vi "PicoScopeospaSettings.vi"(0 "handle in":i16=16384, 1 "Device Info":T3={"PICO_DRIVER_VERSION"="", "PICO_USB_VERSION"="", "PICO_HARDWARE_VERSION"="", "PICO_VARIANT_INFO"="", "PICO_BATCH_AND_SERIAL"="", "PICO_CAL_DATE"="", "PICO_KERNEL_VERSION"="", "PICO_DIGITAL_HARDWARE_VERSION"="", "PICO_ANALOGUE_HARDWARE_VERSION"="", "PICO_FIRMWARE_VERSION_1"="", "PICO_FIRMWARE_VERSION_2"="", "PICO_IPP_VERSION"="", "PICO_DRIVER_PATH"="", "PICO_FIRMWARE_VERSION_3"="", "PICO_FRONT_PANEL_FIRMWARE_VERSION"="", "Number of Channels"=0, "MSO"=TRUE}, 2 "Channels":T2={"Channel A Settings "={"Enabled"=FALSE, "Coupling"=1, "Range"=8, "Analogue Offset"=0.0, "BandWidth"=0, "PROBE_RANGE_INFO"=0}, "Channel B Settings "={"Enabled"=FALSE, "Coupling"=1, "Range"=8, "Analogue Offset"=0.0, "BandWidth"=0, "PROBE_RANGE_INFO"=0}, "Channel C Settings "={"Enabled"=FALSE, "Coupling"=1, "Range"=8, "Analogue Offset"=0.0, "BandWidth"=0, "PROBE_RANGE_INFO"=0}, "Channel D Settings "={"Enabled"=FALSE, "Coupling"=1, "Range"=8, "Analogue Offset"=0.0, "BandWidth"=0, "PROBE_RANGE_INFO"=0}, "Channel E Settings "={"Enabled"=FALSE, "Coupling"=50, "Range"=5, "Analogue Offset"=0.0, "BandWidth"=0, "PROBE_RANGE_INFO"=0}, "Channel F Settings "={"Enabled"=FALSE, "Coupling"=50, "Range"=5, "Analogue Offset"=0.0, "BandWidth"=0, "PROBE_RANGE_INFO"=0}, "Channel G Settings "={"Enabled"=FALSE, "Coupling"=50, "Range"=5, "Analogue Offset"=0.0, "BandWidth"=0, "PROBE_RANGE_INFO"=0}, "Channel H Settings "={"Enabled"=FALSE, "Coupling"=50, "Range"=5, "Analogue Offset"=0.0, "BandWidth"=0, "PROBE_RANGE_INFO"=0}} {"Channel H Settings"."PROBE_RANGE_INFO" items=["PROBE_NONE_NV"=0, "X1_PROBE_NV"=1, "X10_PROBE_NV"=10]; "Channel H Settings"."BandWidth" items=["Full"=0, "100kHz"=100000, "20kHz"=200000, "1MHz"=1000000, "20MHz"=20000000, "25MHz"=25000000, "50MHz"=50000000, "200MHz"=200000000, "250MHz"=250000000, "500MHz"=500000000]; "Channel H Settings"."Range" items=["10mV"=0, "20mV"=1, "50mV"=2, "100mV"=3, "200mV"=4, "500mV"=5, "1V"=6, "2V"=7, "5V"=8, "10V"=9, "20V"=10, "50V"=11, "100V"=12, "200V"=13, "x10_Probe_100mV"=32, "x10_Probe_200mV"=33, "x10_Probe_500mV"=34, "x10_Probe_1V"=35, "x10_Probe_2V"=36, "x10_Probe_5V"=37, "x10_Probe_10V"=38, "x10_Probe_20V"=39, "x10_Probe_50V"=40, "x10_Probe_100V"=41, "x10_Probe_200V"=42, "x10_Probe_500V"=43, "CURRENT_CLAMP_60A_2A"=10500, "CURRENT_CLAMP_60A_5A"=10501, "CURRENT_CLAMP_60A_10A"=10502, "CURRENT_CLAMP_60A_20A"=10503, "CURRENT_CLAMP_60A_50A"=10504, "CURRENT_CLAMP_60A_60A"=10505, "CURRENT_CLAMP_60A_V2_0_5A"=10600, "CURRENT_CLAMP_60A_V2_1A"=10601, "CURRENT_CLAMP_60A_V2_2A"=10602, "CURRENT_CLAMP_60A_V2_5A"=10603, "CURRENT_CLAMP_60A_V2_10A"=10604, "CURRENT_CLAMP_60A_V2_20A"=10605, "CURRENT_CLAMP_60A_V2_50A"=10606, "CURRENT_CLAMP_60A_V2_60A"=10607, "RESISTANCE_LEAD_NEG5_TO_20OHM"=7000, "RESISTANCE_LEAD_NEG50_TO_200OHM"=7001, "RESISTANCE_LEAD_NEG500_TO_2KOHM"=7002, "RESISTANCE_LEAD_NEG5K_TO_20KOHM"=7003, "RESISTANCE_LEAD_NEG50K_TO_LEAD_200KOHM"=7004, "RESISTANCE_LEAD_NEG500K_TO_LEAD_2MOHM"=7005, "RESISTANCE_LEAD_DIODE_TEST"=7006, "HT_NEG3_TO_5KV"=8950, "HT_NEG3_TO_10KV"=8951, "HT_NEG5_TO_20KV"=8952, "HT_NEG5_TO_50KV"=8953, "HT_NEG5_TO_100KV"=8954, "HT_NEG3_TO_5KV_INVERTED"=8955, "HT_NEG3_TO_10KV_INVERTED"=8956, "HT_NEG5_TO_20KV_INVERTED"=8957, "HT_NEG5_TO_50KV_INVERTED"=8958, "HT_NEG5_TO_100KV_INVERTED"=8959, "TEMPERATURE_NEG50_TO_150DEGC"=9000, "PRESSURE_SENSOR_-100k-150k_PASCALS"=9100, "PRESSURE_SENSOR_-100k_TO_400k_PASCALS"=9101, "PRESSURE_SENSOR_-200k_TO_800k_PASCALS"=9102, "PRESSURE_SENSOR_-400k_TO_1600k_PASCALS"=9103, "PRESSURE_SENSOR_-400k_TO_3400k_PASCALS"=9104, "PRESSURE_SENSOR_-150k_TO_1350k_PASCALS"=9105]; "Channel H Settings"."Coupling" items=["AC"=0, "DC 1M Ohm"=1, "DC 50 Ohm"=50]; "Channel G Settings"."PROBE_RANGE_INFO" items=["PROBE_NONE_NV"=0, "X1_PROBE_NV"=1, "X10_PROBE_NV"=10]; "Channel G Settings"."BandWidth" items=["Full"=0, "100kHz"=100000, "20kHz"=200000, "1MHz"=1000000, "20MHz"=20000000, "25MHz"=25000000, "50MHz"=50000000, "200MHz"=200000000, "250MHz"=250000000, "500MHz"=500000000]; "Channel G Settings"."Range" items=["10mV"=0, "20mV"=1, "50mV"=2, "100mV"=3, "200mV"=4, "500mV"=5, "1V"=6, "2V"=7, "5V"=8, "10V"=9, "20V"=10, "50V"=11, "100V"=12, "200V"=13, "x10_Probe_100mV"=32, "x10_Probe_200mV"=33, "x10_Probe_500mV"=34, "x10_Probe_1V"=35, "x10_Probe_2V"=36, "x10_Probe_5V"=37, "x10_Probe_10V"=38, "x10_Probe_20V"=39, "x10_Probe_50V"=40, "x10_Probe_100V"=41, "x10_Probe_200V"=42, "x10_Probe_500V"=43, "CURRENT_CLAMP_60A_2A"=10500, "CURRENT_CLAMP_60A_5A"=10501, "CURRENT_CLAMP_60A_10A"=10502, "CURRENT_CLAMP_60A_20A"=10503, "CURRENT_CLAMP_60A_50A"=10504, "CURRENT_CLAMP_60A_60A"=10505, "CURRENT_CLAMP_60A_V2_0_5A"=10600, "CURRENT_CLAMP_60A_V2_1A"=10601, "CURRENT_CLAMP_60A_V2_2A"=10602, "CURRENT_CLAMP_60A_V2_5A"=10603, "CURRENT_CLAMP_60A_V2_10A"=10604, "CURRENT_CLAMP_60A_V2_20A"=10605, "CURRENT_CLAMP_60A_V2_50A"=10606, "CURRENT_CLAMP_60A_V2_60A"=10607, "RESISTANCE_LEAD_NEG5_TO_20OHM"=7000, "RESISTANCE_LEAD_NEG50_TO_200OHM"=7001, "RESISTANCE_LEAD_NEG500_TO_2KOHM"=7002, "RESISTANCE_LEAD_NEG5K_TO_20KOHM"=7003, "RESISTANCE_LEAD_NEG50K_TO_LEAD_200KOHM"=7004, "RESISTANCE_LEAD_NEG500K_TO_LEAD_2MOHM"=7005, "RESISTANCE_LEAD_DIODE_TEST"=7006, "HT_NEG3_TO_5KV"=8950, "HT_NEG3_TO_10KV"=8951, "HT_NEG5_TO_20KV"=8952, "HT_NEG5_TO_50KV"=8953, "HT_NEG5_TO_100KV"=8954, "HT_NEG3_TO_5KV_INVERTED"=8955, "HT_NEG3_TO_10KV_INVERTED"=8956, "HT_NEG5_TO_20KV_INVERTED"=8957, "HT_NEG5_TO_50KV_INVERTED"=8958, "HT_NEG5_TO_100KV_INVERTED"=8959, "TEMPERATURE_NEG50_TO_150DEGC"=9000, "PRESSURE_SENSOR_-100k-150k_PASCALS"=9100, "PRESSURE_SENSOR_-100k_TO_400k_PASCALS"=9101, "PRESSURE_SENSOR_-200k_TO_800k_PASCALS"=9102, "PRESSURE_SENSOR_-400k_TO_1600k_PASCALS"=9103, "PRESSURE_SENSOR_-400k_TO_3400k_PASCALS"=9104, "PRESSURE_SENSOR_-150k_TO_1350k_PASCALS"=9105]; "Channel G Settings"."Coupling" items=["AC"=0, "DC 1M Ohm"=1, "DC 50 Ohm"=50]; "Channel F Settings"."PROBE_RANGE_INFO" items=["PROBE_NONE_NV"=0, "X1_PROBE_NV"=1, "X10_PROBE_NV"=10]; "Channel F Settings"."BandWidth" items=["Full"=0, "100kHz"=100000, "20kHz"=200000, "1MHz"=1000000, "20MHz"=20000000, "25MHz"=25000000, "50MHz"=50000000, "200MHz"=200000000, "250MHz"=250000000, "500MHz"=500000000]; "Channel F Settings"."Range" items=["10mV"=0, "20mV"=1, "50mV"=2, "100mV"=3, "200mV"=4, "500mV"=5, "1V"=6, "2V"=7, "5V"=8, "10V"=9, "20V"=10, "50V"=11, "100V"=12, "200V"=13, "x10_Probe_100mV"=32, "x10_Probe_200mV"=33, "x10_Probe_500mV"=34, "x10_Probe_1V"=35, "x10_Probe_2V"=36, "x10_Probe_5V"=37, "x10_Probe_10V"=38, "x10_Probe_20V"=39, "x10_Probe_50V"=40, "x10_Probe_100V"=41, "x10_Probe_200V"=42, "x10_Probe_500V"=43, "CURRENT_CLAMP_60A_2A"=10500, "CURRENT_CLAMP_60A_5A"=10501, "CURRENT_CLAMP_60A_10A"=10502, "CURRENT_CLAMP_60A_20A"=10503, "CURRENT_CLAMP_60A_50A"=10504, "CURRENT_CLAMP_60A_60A"=10505, "CURRENT_CLAMP_60A_V2_0_5A"=10600, "CURRENT_CLAMP_60A_V2_1A"=10601, "CURRENT_CLAMP_60A_V2_2A"=10602, "CURRENT_CLAMP_60A_V2_5A"=10603, "CURRENT_CLAMP_60A_V2_10A"=10604, "CURRENT_CLAMP_60A_V2_20A"=10605, "CURRENT_CLAMP_60A_V2_50A"=10606, "CURRENT_CLAMP_60A_V2_60A"=10607, "RESISTANCE_LEAD_NEG5_TO_20OHM"=7000, "RESISTANCE_LEAD_NEG50_TO_200OHM"=7001, "RESISTANCE_LEAD_NEG500_TO_2KOHM"=7002, "RESISTANCE_LEAD_NEG5K_TO_20KOHM"=7003, "RESISTANCE_LEAD_NEG50K_TO_LEAD_200KOHM"=7004, "RESISTANCE_LEAD_NEG500K_TO_LEAD_2MOHM"=7005, "RESISTANCE_LEAD_DIODE_TEST"=7006, "HT_NEG3_TO_5KV"=8950, "HT_NEG3_TO_10KV"=8951, "HT_NEG5_TO_20KV"=8952, "HT_NEG5_TO_50KV"=8953, "HT_NEG5_TO_100KV"=8954, "HT_NEG3_TO_5KV_INVERTED"=8955, "HT_NEG3_TO_10KV_INVERTED"=8956, "HT_NEG5_TO_20KV_INVERTED"=8957, "HT_NEG5_TO_50KV_INVERTED"=8958, "HT_NEG5_TO_100KV_INVERTED"=8959, "TEMPERATURE_NEG50_TO_150DEGC"=9000, "PRESSURE_SENSOR_-100k-150k_PASCALS"=9100, "PRESSURE_SENSOR_-100k_TO_400k_PASCALS"=9101, "PRESSURE_SENSOR_-200k_TO_800k_PASCALS"=9102, "PRESSURE_SENSOR_-400k_TO_1600k_PASCALS"=9103, "PRESSURE_SENSOR_-400k_TO_3400k_PASCALS"=9104, "PRESSURE_SENSOR_-150k_TO_1350k_PASCALS"=9105]; "Channel F Settings"."Coupling" items=["AC"=0, "DC 1M Ohm"=1, "DC 50 Ohm"=50]; "Channel E Settings"."PROBE_RANGE_INFO" items=["PROBE_NONE_NV"=0, "X1_PROBE_NV"=1, "X10_PROBE_NV"=10]; "Channel E Settings"."BandWidth" items=["Full"=0, "100kHz"=100000, "20kHz"=200000, "1MHz"=1000000, "20MHz"=20000000, "25MHz"=25000000, "50MHz"=50000000, "200MHz"=200000000, "250MHz"=250000000, "500MHz"=500000000]; "Channel E Settings"."Range" items=["10mV"=0, "20mV"=1, "50mV"=2, "100mV"=3, "200mV"=4, "500mV"=5, "1V"=6, "2V"=7, "5V"=8, "10V"=9, "20V"=10, "50V"=11, "100V"=12, "200V"=13, "x10_Probe_100mV"=32, "x10_Probe_200mV"=33, "x10_Probe_500mV"=34, "x10_Probe_1V"=35, "x10_Probe_2V"=36, "x10_Probe_5V"=37, "x10_Probe_10V"=38, "x10_Probe_20V"=39, "x10_Probe_50V"=40, "x10_Probe_100V"=41, "x10_Probe_200V"=42, "x10_Probe_500V"=43, "CURRENT_CLAMP_60A_2A"=10500, "CURRENT_CLAMP_60A_5A"=10501, "CURRENT_CLAMP_60A_10A"=10502, "CURRENT_CLAMP_60A_20A"=10503, "CURRENT_CLAMP_60A_50A"=10504, "CURRENT_CLAMP_60A_60A"=10505, "CURRENT_CLAMP_60A_V2_0_5A"=10600, "CURRENT_CLAMP_60A_V2_1A"=10601, "CURRENT_CLAMP_60A_V2_2A"=10602, "CURRENT_CLAMP_60A_V2_5A"=10603, "CURRENT_CLAMP_60A_V2_10A"=10604, "CURRENT_CLAMP_60A_V2_20A"=10605, "CURRENT_CLAMP_60A_V2_50A"=10606, "CURRENT_CLAMP_60A_V2_60A"=10607, "RESISTANCE_LEAD_NEG5_TO_20OHM"=7000, "RESISTANCE_LEAD_NEG50_TO_200OHM"=7001, "RESISTANCE_LEAD_NEG500_TO_2KOHM"=7002, "RESISTANCE_LEAD_NEG5K_TO_20KOHM"=7003, "RESISTANCE_LEAD_NEG50K_TO_LEAD_200KOHM"=7004, "RESISTANCE_LEAD_NEG500K_TO_LEAD_2MOHM"=7005, "RESISTANCE_LEAD_DIODE_TEST"=7006, "HT_NEG3_TO_5KV"=8950, "HT_NEG3_TO_10KV"=8951, "HT_NEG5_TO_20KV"=8952, "HT_NEG5_TO_50KV"=8953, "HT_NEG5_TO_100KV"=8954, "HT_NEG3_TO_5KV_INVERTED"=8955, "HT_NEG3_TO_10KV_INVERTED"=8956, "HT_NEG5_TO_20KV_INVERTED"=8957, "HT_NEG5_TO_50KV_INVERTED"=8958, "HT_NEG5_TO_100KV_INVERTED"=8959, "TEMPERATURE_NEG50_TO_150DEGC"=9000, "PRESSURE_SENSOR_-100k-150k_PASCALS"=9100, "PRESSURE_SENSOR_-100k_TO_400k_PASCALS"=9101, "PRESSURE_SENSOR_-200k_TO_800k_PASCALS"=9102, "PRESSURE_SENSOR_-400k_TO_1600k_PASCALS"=9103, "PRESSURE_SENSOR_-400k_TO_3400k_PASCALS"=9104, "PRESSURE_SENSOR_-150k_TO_1350k_PASCALS"=9105]; "Channel E Settings"."Coupling" items=["AC"=0, "DC 1M Ohm"=1, "DC 50 Ohm"=50]; "Channel D Settings"."BandWidth" items=["Full"=0, "100kHz"=100000, "20kHz"=200000, "1MHz"=1000000, "20MHz"=20000000, "25MHz"=25000000, "50MHz"=50000000, "100MHz"=100000000, "200MHz"=200000000, "250MHz"=250000000, "350MHz"=350000000, "500MHz"=500000000]; "Channel D Settings"."PROBE_RANGE_INFO" items=["PROBE_NONE_NV"=0, "X1_PROBE_NV"=1, "X10_PROBE_NV"=10]; "Channel D Settings"."Range" items=["10mV", "20mV", "50mV", "100mV", "200mV", "500mV", "1V", "2V", "5V", "10V", "20V", "50V", "100V", "200V"]; "Channel D Settings"."Coupling" items=["AC"=0, "DC 1M Ohm"=1, "DC 50 Ohm"=50]; "Channel C Settings"."BandWidth" items=["Full"=0, "100kHz"=100000, "20kHz"=200000, "1MHz"=1000000, "20MHz"=20000000, "25MHz"=25000000, "50MHz"=50000000, "100MHz"=100000000, "200MHz"=200000000, "250MHz"=250000000, "350MHz"=350000000, "500MHz"=500000000]; "Channel C Settings"."PROBE_RANGE_INFO" items=["PROBE_NONE_NV"=0, "X1_PROBE_NV"=1, "X10_PROBE_NV"=10]; "Channel C Settings"."Range" items=["10mV", "20mV", "50mV", "100mV", "200mV", "500mV", "1V", "2V", "5V", "10V", "20V", "50V", "100V", "200V"]; "Channel C Settings"."Coupling" items=["AC"=0, "DC 1M Ohm"=1, "DC 50 Ohm"=50]; "Channel B Settings"."BandWidth" items=["Full"=0, "100kHz"=100000, "20kHz"=200000, "1MHz"=1000000, "20MHz"=20000000, "25MHz"=25000000, "50MHz"=50000000, "100MHz"=100000000, "200MHz"=200000000, "250MHz"=250000000, "350MHz"=350000000, "500MHz"=500000000]; "Channel B Settings"."PROBE_RANGE_INFO" items=["PROBE_NONE_NV"=0, "X1_PROBE_NV"=1, "X10_PROBE_NV"=10]; "Channel B Settings"."Range" items=["10mV", "20mV", "50mV", "100mV", "200mV", "500mV", "1V", "2V", "5V", "10V", "20V", "50V", "100V", "200V"]; "Channel B Settings"."Coupling" items=["AC"=0, "DC 1M Ohm"=1, "DC 50 Ohm"=50]; "Channel A Settings"."PROBE_RANGE_INFO" items=["PROBE_NONE_NV"=0, "X1_PROBE_NV"=1, "X10_PROBE_NV"=10]; "Channel A Settings"."Range" items=["10mV", "20mV", "50mV", "100mV", "200mV", "500mV", "1V", "2V", "5V", "10V", "20V", "50V", "100V", "200V"]; "Channel A Settings"."BandWidth" items=["Full"=0, "100kHz"=100000, "20kHz"=200000, "1MHz"=1000000, "20MHz"=20000000, "25MHz"=25000000, "50MHz"=50000000, "100MHz"=100000000, "200MHz"=200000000, "250MHz"=250000000, "350MHz"=350000000, "500MHz"=500000000]; "Channel A Settings"."Coupling" items=["AC"=0, "DC 1M Ohm"=1, "DC 50 Ohm"=50]}, 7 "Max ADC value":i16=32512, 11 "error in (no error)":errorcluster, 12 "Trigger Settings":T4={"Trigger Enabled"=FALSE, "Trigger Threshold (Volts/Probe Units)"=0.0, "Trigger Direction"=2, "Trigger Delay (samples)"=0, "Auto Trigger Time (us)"=1000000, "Trigger Source"=0} {"Trigger Source" items=["Channel A"=0, "Channel B"=1, "Channel C"=2, "Channel D"=3, "Channel E"=4, "Channel F"=5, "Channel G"=6, "Channel H"=7, "Port 0"=128, "Port 1"=129, "Trigger AUX"=1001]; "Trigger Direction" items=["Above", "Below", "Rising", "Falling", "Rising or Falling"]; "Trigger Threshold (Volts/Probe Units)" format="%#_6p"}, 14 "Digital Channels":T1 {"Port 1 Settings"."Threshold Level (Volts)" format="%#_4p"; "Port 0 Settings"."Threshold Level (Volts)" format="%#_4p"}) -> (3 "Enabled array":i16[](array[numeric])=[1, 0, 0, 0, 0, 0, 0, 0, 0, 0], 4 "handle out":i16=16384, 15 "error out":errorcluster)   [LabVIEW 2024]
doc: "Sets up channels and calls setSimpleTrigger"
uses:
  PicoScopeospaAnalogChannelSettings.ctl
  PicoScopeospaDigitalChannelSettings.ctl
  psospa.dll
panel:
  # "D8-D15"
  # "DO-D7"
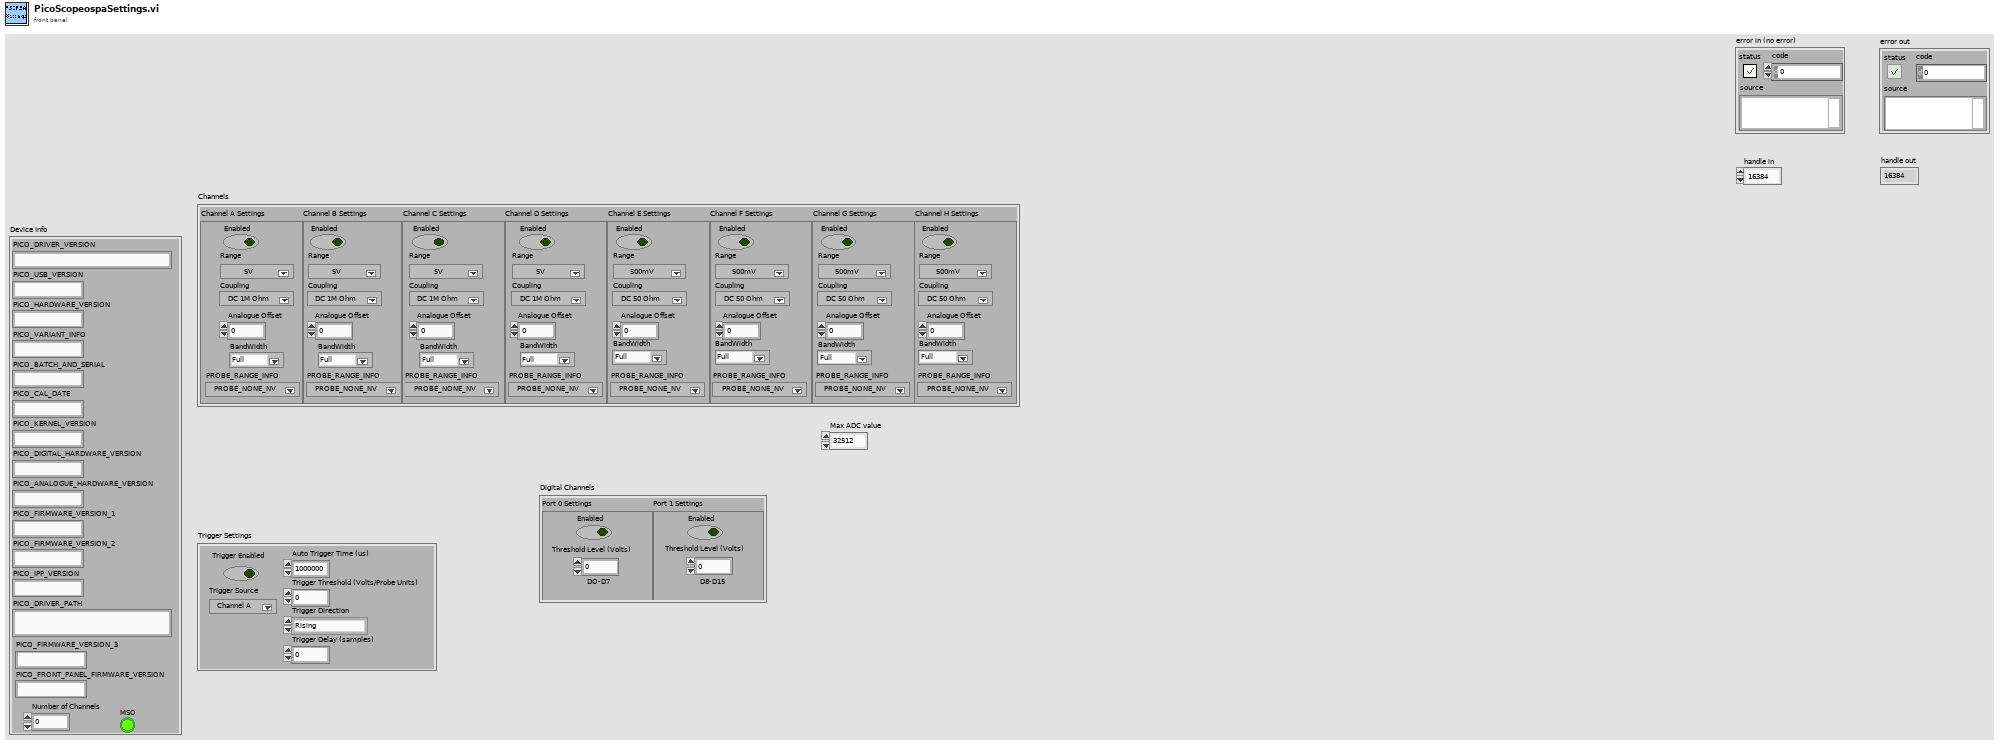
[diagram p1: front panel]
types:
  T1 = typedef "PicoScopeospaDigitalChannelSettings.ctl" = cluster{"Port 0 Settings ":cluster{"Enabled":bool, "Threshold Level (Volts)":dbl}, "Port 1 Settings":cluster{"Enabled":bool, "Threshold Level (Volts)":dbl}}
  T2 = typedef "PicoScopeospaAnalogChannelSettings.ctl" = cluster{"Channel A Settings ":cluster{"Enabled":bool, "Coupling":i16, "Range":u16, "Analogue Offset":dbl, "BandWidth":u32, "PROBE_RANGE_INFO":u32}, "Channel B Settings ":cluster{"Enabled":bool, "Coupling":i16, "Range":u16, "Analogue Offset":dbl, "BandWidth":u32, "PROBE_RANGE_INFO":u32}, "Channel C Settings ":cluster{"Enabled":bool, "Coupling":i16, "Range":u16, "Analogue Offset":dbl, "BandWidth":u32, "PROBE_RANGE_INFO":u32}, "Channel D Settings ":cluster{"Enabled":bool, "Coupling":i16, "Range":u16, "Analogue Offset":dbl, "BandWidth":u32, "PROBE_RANGE_INFO":u32}, "Channel E Settings ":cluster{"Enabled":bool, "Coupling":i16, "Range":u16, "Analogue Offset":dbl, "BandWidth":u32, "PROBE_RANGE_INFO":u32}, "Channel F Settings ":cluster{"Enabled":bool, "Coupling":i16, "Range":u16, "Analogue Offset":dbl, "BandWidth":u32, "PROBE_RANGE_INFO":u32}, "Channel G Settings ":cluster{"Enabled":bool, "Coupling":i16, "Range":u16, "Analogue Offset":dbl, "BandWidth":u32, "PROBE_RANGE_INFO":u32}, "Channel H Settings ":cluster{"Enabled":bool, "Coupling":i16, "Range":u16, "Analogue Offset":dbl, "BandWidth":u32, "PROBE_RANGE_INFO":u32}}
  T3 = cluster{"PICO_DRIVER_VERSION":string, "PICO_USB_VERSION":string, "PICO_HARDWARE_VERSION":string, "PICO_VARIANT_INFO":string, "PICO_BATCH_AND_SERIAL":string, "PICO_CAL_DATE":string, "PICO_KERNEL_VERSION":string, "PICO_DIGITAL_HARDWARE_VERSION":string, "PICO_ANALOGUE_HARDWARE_VERSION":string, "PICO_FIRMWARE_VERSION_1":string, "PICO_FIRMWARE_VERSION_2":string, "PICO_IPP_VERSION":string, "PICO_DRIVER_PATH":string, "PICO_FIRMWARE_VERSION_3":string, "PICO_FRONT_PANEL_FIRMWARE_VERSION":string, "Number of Channels":i16, "MSO":bool}
  T4 = cluster{"Trigger Enabled":bool, "Trigger Threshold (Volts/Probe Units)":dbl, "Trigger Direction":u16, "Trigger Delay (samples)":u64, "Auto Trigger Time (us)":u32, "Trigger Source":u32}
  T5 = cluster{"Enabled":bool, "Coupling":i16, "Range":u16, "Analogue Offset":dbl, "BandWidth":u32, "PROBE_RANGE_INFO":u32}
  T6 = cluster{"Enabled":bool, "Threshold Level (Volts)":dbl}
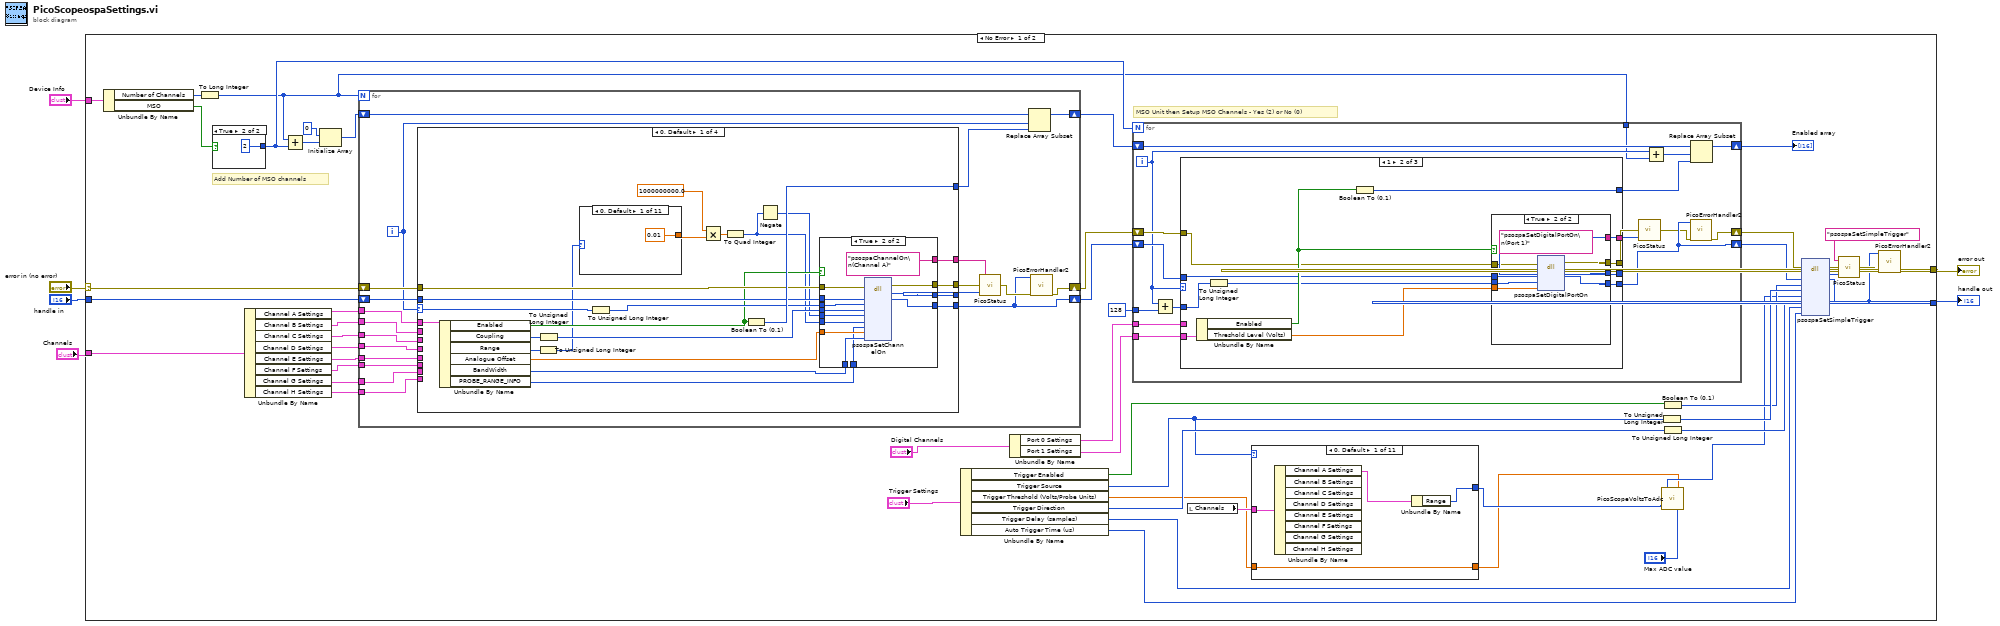
[diagram p0: block diagram]
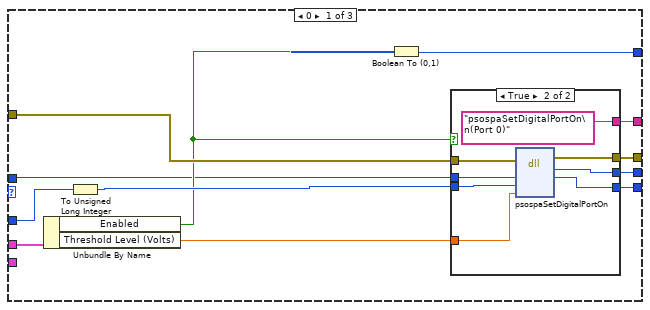
[diagram p2: hidden frame]
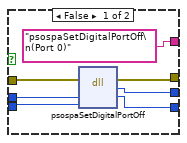
[diagram p3: hidden frame]
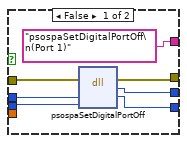
[diagram p4: hidden frame]
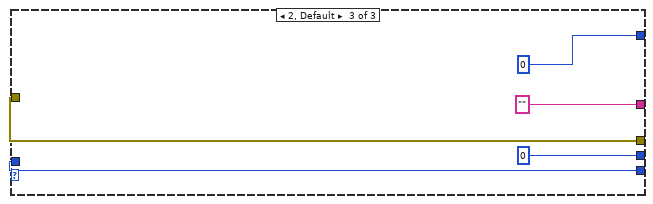
[diagram p5: hidden frame]
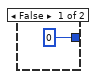
[diagram p6: hidden frame]
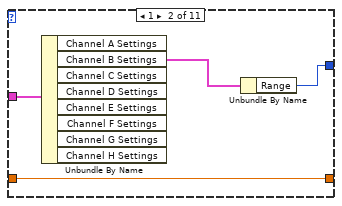
[diagram p7: hidden frame]
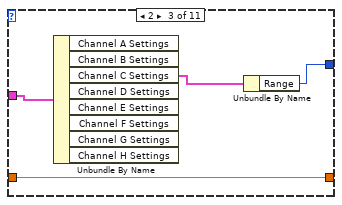
[diagram p8: hidden frame]
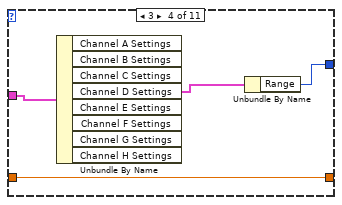
[diagram p9: hidden frame]
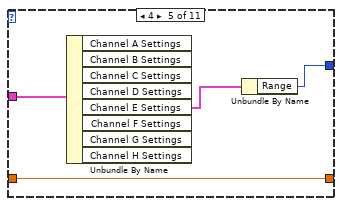
[diagram p10: hidden frame]
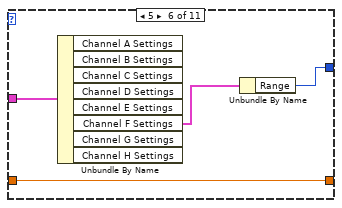
[diagram p11: hidden frame]
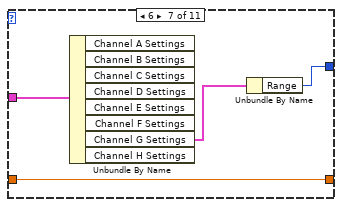
[diagram p12: hidden frame]
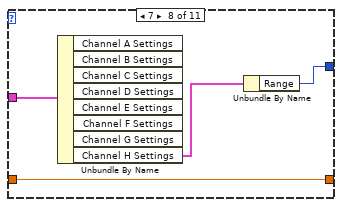
[diagram p13: hidden frame]
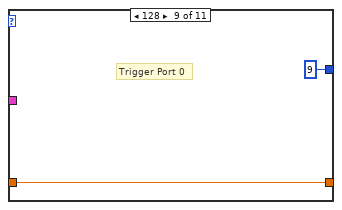
[diagram p14: hidden frame]
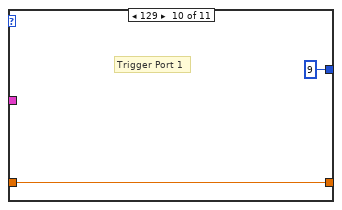
[diagram p15: hidden frame]
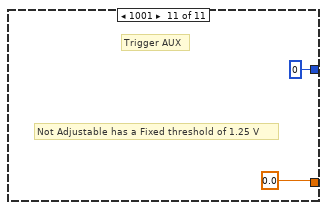
[diagram p16: hidden frame]
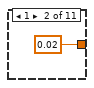
[diagram p17: hidden frame]
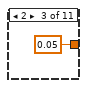
[diagram p18: hidden frame]
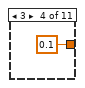
[diagram p19: hidden frame]
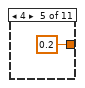
[diagram p20: hidden frame]
diagram:
  n1 = case shown="No Error" "error in (no error)" {
    selector: "error in (no error)" -> [w44 w411]
    tunnel: "handle in" -> [w45 w410]
    tunnel: [w37 w410] -> w6
    tunnel: [w39 w411] -> w5
    tunnel: "Device Info" -> [w41 _]
    tunnel: "Channels" -> [w28 _]
    frame No Error {
      # "Add Number of MSO channels"
      # "MSO Unit then Setup MSO Channels - Yes (2) or No (0)"
      n2 = Unbundle By Name(w41) -> ("Number of Channels"=w40:i16, "MSO"=w11:bool)
      n3 = To Long Integer(number=w40) -> (32bit integer=w8:i32)
      n4 = case shown="True" w11 {
        tunnel: [0 ("y") 2 ("y")] -> w9
        frame False {
        }
        frame True {
        }
      }
      n5 = Unbundle By Name(w28) -> ("Channel A Settings"=w35:T5, "Channel B Settings"=w36:T5, "Channel C Settings"=w34:T5, "Channel D Settings"=w33:T5, "Channel E Settings"=w32:T5, "Channel F Settings"=w29:T5, "Channel G Settings"=w30:T5, "Channel H Settings"=w31:T5)
      n6 = Add(x=w8, y=w9) -> (x+y=w12:i32)
      n7 = Initialize Array(i16 0 ("element"), w12) -> (w42:i16[])
      n8 = for {
        N: w8 -> [_]
        shift-right: [w187] -> w24
        shift-left: w44 -> [w192]
        shift-right: [w182] -> w23
        shift-left: w45 -> [w193]
        shift-right: [w188] -> w26
        shift-left: w42 -> [w189]
        tunnel: w36 -> [w181]
        tunnel: w35 -> [w180]
        tunnel: w34 -> [w179]
        tunnel: w33 -> [w178]
        tunnel: w32 -> [w177]
        tunnel: w31 -> [w176]
        tunnel: w30 -> [w175]
        tunnel: w29 -> [w174]
        i -> [w191]
        n9 = case shown="0, Default" w191 {
          selector: w191 -> [w216 w270 w324 w378]
          tunnel: w193 -> [w209 w263 w317 w371]
          tunnel: w192 -> [w211 w265 w319 w373]
          tunnel: [w213 w267 w321 w375] -> w190
          tunnel: [w204 w258 w312 w366] -> w186
          tunnel: [w210 w264 w318 w372] -> w185
          tunnel: [w212 w266 w320 w374] -> w184
          tunnel: [w203 w257 w311 w365] -> w182
          tunnel: w181 -> [_ w248 _ _]
          tunnel: w180 -> [w202 _ _ _]
          tunnel: w179 -> [_ _ w302 _]
          tunnel: w178 -> [_ _ _ w356]
          tunnel: w177 -> [_ _ _ _]
          tunnel: w176 -> [_ _ _ _]
          tunnel: w175 -> [_ _ _ _]
          tunnel: w174 -> [_ _ _ _]
          frame 0, Default {
            n10 = Unbundle By Name(w202) -> ("Enabled"=w205:bool, "Coupling"=w215:i16, "Range"=w214:u16, "Analogue Offset"=w206:dbl, "BandWidth"=w201:u32, "PROBE_RANGE_INFO"=w197:u32)
            n11 = To Unsigned Long Integer(number=w214) -> (unsigned 32bit integer=w200:u32)
            n12 = To Unsigned Long Integer(number=w215) -> (unsigned 32bit integer=w207:u32)
            n13 = case shown="0, Default" w200 {
              tunnel: [0.01 ("rangeMin") 0.02 ("rangeMin") 0.05 ("rangeMin") 0.1 ("rangeMin") 0.2 ("rangeMin") 0.5 ("rangeMin") 1.0 ("rangeMin") 2.0 ("rangeMin") 5.0 ("rangeMin") 10.0 ("rangeMin") 20.0 ("rangeMin")] -> w199
              frame 0, Default {
              }
              frame 1 {
              }
              frame 2 {
              }
              frame 3 {
              }
              frame 4 {
              }
              frame 5 {
              }
              frame 6 {
              }
              frame 7 {
              }
              frame 8 {
              }
              frame 9 {
              }
              frame 10 {
              }
            }
            n14 = To Unsigned Long Integer(number=w216) -> (unsigned 32bit integer=w208:u32)
            n15 = Multiply(x=1000000000.0, y=w199) -> (x*y=w198:dbl)
            n16 = To Quad Integer(1:w198) -> (0:w195:i64)
            n17 = Boolean To (0,1)(Boolean=w205) -> (0, 1=w213:i16)
            n18 = Negate(x=w195) -> (-x=w196:i64)
            n19 = case shown="True" w205 {
              tunnel: ["psospaSetChannelOff\n(Channel A)" ("source") "psospaChannelOn\n(Channel A)" ("source")] -> w212
              tunnel: w211 -> [w233 w246]
              tunnel: [w232 w245] -> w210
              tunnel: w209 -> [w231 w244]
              tunnel: w208 -> [w230 w243]
              tunnel: w207 -> [_ w242]
              tunnel: w206 -> [_ w241]
              tunnel: [w229 w240] -> w204
              tunnel: [w228 w239] -> w203
              tunnel: w201 -> [_ w238]
              tunnel: w197 -> [_ w237]
              tunnel: w196 -> [_ w235]
              tunnel: w195 -> [_ w236]
              frame False {
                n20 = dll-call lib="psospa.dll" fn="psospaSetChannelOff" ("ps3000.dll:_ps3000_open_unit@0")(error in=w233, "handle"=w231, "channel"=w230) -> (error out=w232:errorcluster, "PICO_STATUS"=w229:u32, "handle"=w228:i16)  [unwired: 3 in, 1 out]
              }
              frame True {
                n21 = dll-call lib="psospa.dll" fn="psospaSetChannelOn" ("ps3000.dll:_ps3000_open_unit@0")(error in=w246, "handle"=w244, "channel"=w243, "coupling"=w242, "rangeMin"=w235, "rangeMax"=w236, "rangeType"=w237, "analogueOffset"=w241, "bandwidth"=w238) -> (error out=w245:errorcluster, "PICO_STATUS"=w240:u32, "handle"=w239:i16)  [unwired: 9 in, 1 out]
              }
            }
          }
          frame 1 {
            n22 = Unbundle By Name(w248) -> ("Enabled"=w259:bool, "Coupling"=w269:i16, "Range"=w268:u16, "Analogue Offset"=w260:dbl, "BandWidth"=w256:u32, "PROBE_RANGE_INFO"=w252:u32)
            n23 = To Unsigned Long Integer(number=w268) -> (unsigned 32bit integer=w255:u32)
            n24 = To Unsigned Long Integer(number=w269) -> (unsigned 32bit integer=w261:u32)
            n25 = case shown="9" w255 {
              tunnel: [0.01 ("rangeMin") 0.02 ("rangeMin") 0.05 ("rangeMin") 0.1 ("rangeMin") 0.2 ("rangeMin") 0.5 ("rangeMin") 1.0 ("rangeMin") 2.0 ("rangeMin") 5.0 ("rangeMin") 10.0 ("rangeMin") 20.0 ("rangeMin")] -> w254
              frame 0, Default {
              }
              frame 1 {
              }
              frame 2 {
              }
              frame 3 {
              }
              frame 4 {
              }
              frame 5 {
              }
              frame 6 {
              }
              frame 7 {
              }
              frame 8 {
              }
              frame 9 {
              }
              frame 10 {
              }
            }
            n26 = To Unsigned Long Integer(number=w270) -> (unsigned 32bit integer=w262:u32)
            n27 = Multiply(x=1000000000.0, y=w254) -> (x*y=w253:dbl)
            n28 = To Quad Integer(1:w253) -> (0:w250:i64)
            n29 = Boolean To (0,1)(Boolean=w259) -> (0, 1=w267:i16)
            n30 = Negate(x=w250) -> (-x=w251:i64)
            n31 = case shown="False" w259 {
              tunnel: ["psospaSetChannelOff\n(Channel B)" ("source") "psospaChannelOn\n(Channel B)" ("source")] -> w266
              tunnel: w265 -> [w287 w300]
              tunnel: [w286 w299] -> w264
              tunnel: w263 -> [w285 w298]
              tunnel: w262 -> [w284 w297]
              tunnel: w261 -> [_ w296]
              tunnel: w260 -> [_ w295]
              tunnel: [w283 w294] -> w258
              tunnel: [w282 w293] -> w257
              tunnel: w256 -> [_ w292]
              tunnel: w252 -> [_ w291]
              tunnel: w251 -> [_ w289]
              tunnel: w250 -> [_ w290]
              frame False {
                n32 = dll-call lib="psospa.dll" fn="psospaSetChannelOff" ("ps3000.dll:_ps3000_open_unit@0")(error in=w287, "handle"=w285, "channel"=w284) -> (error out=w286:errorcluster, "PICO_STATUS"=w283:u32, "handle"=w282:i16)  [unwired: 3 in, 1 out]
              }
              frame True {
                n33 = dll-call lib="psospa.dll" fn="psospaSetChannelOn" ("ps3000.dll:_ps3000_open_unit@0")(error in=w300, "handle"=w298, "channel"=w297, "coupling"=w296, "rangeMin"=w289, "rangeMax"=w290, "rangeType"=w291, "analogueOffset"=w295, "bandwidth"=w292) -> (error out=w299:errorcluster, "PICO_STATUS"=w294:u32, "handle"=w293:i16)  [unwired: 9 in, 1 out]
              }
            }
          }
          frame 2 {
            n34 = Unbundle By Name(w302) -> ("Enabled"=w313:bool, "Coupling"=w323:i16, "Range"=w322:u16, "Analogue Offset"=w314:dbl, "BandWidth"=w310:u32, "PROBE_RANGE_INFO"=w306:u32)
            n35 = To Unsigned Long Integer(number=w322) -> (unsigned 32bit integer=w309:u32)
            n36 = To Unsigned Long Integer(number=w323) -> (unsigned 32bit integer=w315:u32)
            n37 = case shown="8" w309 {
              tunnel: [0.01 ("rangeMin") 0.02 ("rangeMin") 0.05 ("rangeMin") 0.1 ("rangeMin") 0.2 ("rangeMin") 0.5 ("rangeMin") 1.0 ("rangeMin") 2.0 ("rangeMin") 5.0 ("rangeMin") 10.0 ("rangeMin") 20.0 ("rangeMin")] -> w308
              frame 0, Default {
              }
              frame 1 {
              }
              frame 2 {
              }
              frame 3 {
              }
              frame 4 {
              }
              frame 5 {
              }
              frame 6 {
              }
              frame 7 {
              }
              frame 8 {
              }
              frame 9 {
              }
              frame 10 {
              }
            }
            n38 = To Unsigned Long Integer(number=w324) -> (unsigned 32bit integer=w316:u32)
            n39 = Multiply(x=1000000000.0, y=w308) -> (x*y=w307:dbl)
            n40 = To Quad Integer(1:w307) -> (0:w304:i64)
            n41 = Boolean To (0,1)(Boolean=w313) -> (0, 1=w321:i16)
            n42 = Negate(x=w304) -> (-x=w305:i64)
            n43 = case shown="True" w313 {
              tunnel: ["psospaSetChannelOff\n(Channel C)" ("source") "psospaChannelOn\n(Channel C)" ("source")] -> w320
              tunnel: w319 -> [w341 w354]
              tunnel: [w340 w353] -> w318
              tunnel: w317 -> [w339 w352]
              tunnel: w316 -> [w338 w351]
              tunnel: w315 -> [_ w350]
              tunnel: w314 -> [_ w349]
              tunnel: [w337 w348] -> w312
              tunnel: [w336 w347] -> w311
              tunnel: w310 -> [_ w346]
              tunnel: w306 -> [_ w345]
              tunnel: w305 -> [_ w343]
              tunnel: w304 -> [_ w344]
              frame False {
                n44 = dll-call lib="psospa.dll" fn="psospaSetChannelOff" ("ps3000.dll:_ps3000_open_unit@0")(error in=w341, "handle"=w339, "channel"=w338) -> (error out=w340:errorcluster, "PICO_STATUS"=w337:u32, "handle"=w336:i16)  [unwired: 3 in, 1 out]
              }
              frame True {
                n45 = dll-call lib="psospa.dll" fn="psospaSetChannelOn" ("ps3000.dll:_ps3000_open_unit@0")(error in=w354, "handle"=w352, "channel"=w351, "coupling"=w350, "rangeMin"=w343, "rangeMax"=w344, "rangeType"=w345, "analogueOffset"=w349, "bandwidth"=w346) -> (error out=w353:errorcluster, "PICO_STATUS"=w348:u32, "handle"=w347:i16)  [unwired: 9 in, 1 out]
              }
            }
          }
          frame 3 {
            n46 = Unbundle By Name(w356) -> ("Enabled"=w367:bool, "Coupling"=w377:i16, "Range"=w376:u16, "Analogue Offset"=w368:dbl, "BandWidth"=w364:u32, "PROBE_RANGE_INFO"=w360:u32)
            n47 = To Unsigned Long Integer(number=w376) -> (unsigned 32bit integer=w363:u32)
            n48 = To Unsigned Long Integer(number=w377) -> (unsigned 32bit integer=w369:u32)
            n49 = case shown="8" w363 {
              tunnel: [0.01 ("rangeMin") 0.02 ("rangeMin") 0.05 ("rangeMin") 0.1 ("rangeMin") 0.2 ("rangeMin") 0.5 ("rangeMin") 1.0 ("rangeMin") 2.0 ("rangeMin") 5.0 ("rangeMin") 10.0 ("rangeMin") 20.0 ("rangeMin")] -> w362
              frame 0, Default {
              }
              frame 1 {
              }
              frame 2 {
              }
              frame 3 {
              }
              frame 4 {
              }
              frame 5 {
              }
              frame 6 {
              }
              frame 7 {
              }
              frame 8 {
              }
              frame 9 {
              }
              frame 10 {
              }
            }
            n50 = To Unsigned Long Integer(number=w378) -> (unsigned 32bit integer=w370:u32)
            n51 = Multiply(x=1000000000.0, y=w362) -> (x*y=w361:dbl)
            n52 = To Quad Integer(1:w361) -> (0:w358:i64)
            n53 = Boolean To (0,1)(Boolean=w367) -> (0, 1=w375:i16)
            n54 = Negate(x=w358) -> (-x=w359:i64)
            n55 = case shown="True" w367 {
              tunnel: ["psospaSetChannelOff\n(Channel D)" ("source") "psospaChannelOn\n(Channel D)" ("source")] -> w374
              tunnel: w373 -> [w395 w408]
              tunnel: [w394 w407] -> w372
              tunnel: w371 -> [w393 w406]
              tunnel: w370 -> [w392 w405]
              tunnel: w369 -> [_ w404]
              tunnel: w368 -> [_ w403]
              tunnel: [w391 w402] -> w366
              tunnel: [w390 w401] -> w365
              tunnel: w364 -> [_ w400]
              tunnel: w360 -> [_ w399]
              tunnel: w359 -> [_ w397]
              tunnel: w358 -> [_ w398]
              frame False {
                n56 = dll-call lib="psospa.dll" fn="psospaSetChannelOff" ("ps3000.dll:_ps3000_open_unit@0")(error in=w395, "handle"=w393, "channel"=w392) -> (error out=w394:errorcluster, "PICO_STATUS"=w391:u32, "handle"=w390:i16)  [unwired: 3 in, 1 out]
              }
              frame True {
                n57 = dll-call lib="psospa.dll" fn="psospaSetChannelOn" ("ps3000.dll:_ps3000_open_unit@0")(error in=w408, "handle"=w406, "channel"=w405, "coupling"=w404, "rangeMin"=w397, "rangeMax"=w398, "rangeType"=w399, "analogueOffset"=w403, "bandwidth"=w400) -> (error out=w407:errorcluster, "PICO_STATUS"=w402:u32, "handle"=w401:i16)  [unwired: 9 in, 1 out]
              }
            }
          }
        }
        n58 = call "PicoStatus.vi"("PICO STATUS"=w186, "error in"=w185, "source"=w184) -> ("error out"=w183:errorcluster)
        n59 = Replace Array Subset(array=w189, new element=w190, index=w191) -> (w188:i16[])
        n60 = call "PicoErrorHandler2.vi"("error in (no error)"=w183, "handle In"=w182) -> ("error out"=w187:errorcluster)  [unwired: 9 in]
      }
      n61 = Unbundle By Name("Trigger Settings") -> ("Trigger Enabled"=w50:bool, "Trigger Source"=w16:u32, "Trigger Threshold (Volts/Probe Units)"=w15:dbl, "Trigger Direction"=w53:u16, "Trigger Delay (samples)"=w52:u64, "Auto Trigger Time (us)"=w51:u32)
      n62 = Unbundle By Name("Digital Channels") -> ("Port 0 Settings"=w25:T6, "Port 1 Settings"=w20:T6)
      n63 = for {
        N: w9 -> [_]
        shift-right: [w69] -> w22
        shift-left: w24 -> [w73]
        shift-right: [w65] -> w21
        shift-left: w23 -> [w74]
        shift-right: [w70] -> w27
        shift-left: w26 -> [w71]
        tunnel: w25 -> [w64]
        tunnel: 128 -> [w61]
        tunnel: w20 -> [w59]
        tunnel: w8 -> [w57]
        i -> [w60]
        n64 = Add(x=w60, y=w61) -> (x+y=w62:i32)
        n65 = case shown="1" w60 {
          tunnel: w74 -> [w78 w103 w132]
          tunnel: w73 -> [w84 w105 w133]
          tunnel: [w86 w113 i16 0] -> w72
          tunnel: [w81 w110 u32 0 ("PICO_STATUS")] -> w68
          tunnel: [w83 w111 w133] -> w67
          tunnel: [w85 w112 "" ("source")] -> w66
          tunnel: [w80 w109 w132] -> w65
          tunnel: w64 -> [w76 _ _]
          tunnel: w62 -> [w77 w108 _]
          tunnel: w59 -> [_ w107 _]
          frame 0 {
            n66 = Unbundle By Name(w76) -> ("Enabled"=w79:bool, "Threshold Level (Volts)"=w75:dbl)
            n67 = To Unsigned Long Integer(number=w77) -> (unsigned 32bit integer=w82:u32)
            n68 = Boolean To (0,1)(Boolean=w79) -> (0, 1=w86:i16)
            n69 = case shown="True" w79 {
              tunnel: ["psospaSetDigitalPortOff\n(Port 0)" ("source") "psospaSetDigitalPortOn\n(Port 0)" ("source")] -> w85
              tunnel: w84 -> [w92 w100]
              tunnel: [w91 w99] -> w83
              tunnel: w82 -> [w90 w98]
              tunnel: [w89 w97] -> w81
              tunnel: [w88 w96] -> w80
              tunnel: w78 -> [w87 w95]
              tunnel: w75 -> [_ w94]
              frame False {
                n70 = dll-call lib="psospa.dll" fn="psospaSetDigitalPortOff" ("ps3000.dll:_ps3000_open_unit@0")(error in=w92, "handle"=w87, "port"=w90) -> (error out=w91:errorcluster, "PICO_STATUS"=w89:u32, "handle"=w88:i16)  [unwired: 3 in, 1 out]
              }
              frame True {
                n71 = dll-call lib="psospa.dll" fn="psospaSetDigitalPortOn" ("ps3000.dll:_ps3000_open_unit@0")(error in=w100, "handle"=w95, "port"=w98, "logicThresholdLevel"=w94) -> (error out=w99:errorcluster, "PICO_STATUS"=w97:u32, "handle"=w96:i16)  [unwired: 4 in, 1 out]
              }
            }
          }
          frame 1 {
            n72 = Unbundle By Name(w107) -> ("Enabled"=w106:bool, "Threshold Level (Volts)"=w102:dbl)
            n73 = To Unsigned Long Integer(number=w108) -> (unsigned 32bit integer=w104:u32)
            n74 = Boolean To (0,1)(Boolean=w106) -> (0, 1=w113:i16)
            n75 = case shown="True" w106 {
              tunnel: ["psospaSetDigitalPortOff\n(Port 1)" ("source") "psospaSetDigitalPortOn\n(Port 1)" ("source")] -> w112
              tunnel: w105 -> [w119 w127]
              tunnel: [w118 w126] -> w111
              tunnel: w104 -> [w117 w125]
              tunnel: w102 -> [_ w121]
              tunnel: [w116 w124] -> w110
              tunnel: [w115 w123] -> w109
              tunnel: w103 -> [w114 w122]
              frame False {
                n76 = dll-call lib="psospa.dll" fn="psospaSetDigitalPortOff" ("ps3000.dll:_ps3000_open_unit@0")(error in=w119, "handle"=w114, "port"=w117) -> (error out=w118:errorcluster, "PICO_STATUS"=w116:u32, "handle"=w115:i16)  [unwired: 3 in, 1 out]
              }
              frame True {
                n77 = dll-call lib="psospa.dll" fn="psospaSetDigitalPortOn" ("ps3000.dll:_ps3000_open_unit@0")(error in=w127, "handle"=w122, "port"=w125, "logicThresholdLevel"=w121) -> (error out=w126:errorcluster, "PICO_STATUS"=w124:u32, "handle"=w123:i16)  [unwired: 4 in, 1 out]
              }
            }
          }
          frame 2, Default {
          }
        }
        n78 = call "PicoStatus.vi"("PICO STATUS"=w68, "error in"=w67, "source"=w66) -> ("error out"=w63:errorcluster)
        n79 = Add(x=w60, y=w57) -> (x+y=w58:i32)
        n80 = call "PicoErrorHandler2.vi"("error in (no error)"=w63, "handle In"=w65) -> ("error out"=w69:errorcluster)  [unwired: 9 in]
        n81 = Replace Array Subset(array=w71, new element=w72, index=w58) -> (w70:i16[])
      }
      "Enabled array" <- w27
      n82 = local read "Channels"() -> (w19:T2)
      n83 = case shown="0, Default" w16 {
        tunnel: [w139 w143 w147 w151 w155 w159 w163 w167 u16 9 ("Range") u16 9 ("Range") u16 0 ("Range")] -> w14
        tunnel: w19 -> [w138 w142 w146 w150 w154 w158 w162 w166 _ _ _]
        tunnel: w15 -> [w136 w140 w144 w148 w152 w156 w160 w164 w168 w170 _]
        tunnel: [w136 w140 w144 w148 w152 w156 w160 w164 w168 w170 0.0 ("Trigger Threshold (Volts/Probe Units)")] -> w13
        frame 0, Default {
          n84 = Unbundle By Name(w138) -> ("Channel A Settings"=w137:T5)  [unwired: 7 out]
          n85 = Unbundle By Name(w137) -> ("Range"=w139:u16)
        }
        frame 1 {
          n86 = Unbundle By Name(w142) -> ("Channel B Settings"=w141:T5)  [unwired: 7 out]
          n87 = Unbundle By Name(w141) -> ("Range"=w143:u16)
        }
        frame 2 {
          n88 = Unbundle By Name(w146) -> ("Channel C Settings"=w145:T5)  [unwired: 7 out]
          n89 = Unbundle By Name(w145) -> ("Range"=w147:u16)
        }
        frame 3 {
          n90 = Unbundle By Name(w150) -> ("Channel D Settings"=w149:T5)  [unwired: 7 out]
          n91 = Unbundle By Name(w149) -> ("Range"=w151:u16)
        }
        frame 4 {
          n92 = Unbundle By Name(w154) -> ("Channel E Settings"=w153:T5)  [unwired: 7 out]
          n93 = Unbundle By Name(w153) -> ("Range"=w155:u16)
        }
        frame 5 {
          n94 = Unbundle By Name(w158) -> ("Channel F Settings"=w157:T5)  [unwired: 7 out]
          n95 = Unbundle By Name(w157) -> ("Range"=w159:u16)
        }
        frame 6 {
          n96 = Unbundle By Name(w162) -> ("Channel G Settings"=w161:T5)  [unwired: 7 out]
          n97 = Unbundle By Name(w161) -> ("Range"=w163:u16)
        }
        frame 7 {
          n98 = Unbundle By Name(w166) -> ("Channel H Settings"=w165:T5)  [unwired: 7 out]
          n99 = Unbundle By Name(w165) -> ("Range"=w167:u16)
        }
        frame 128 {
          # "Trigger Port 0"
        }
        frame 129 {
          # "Trigger Port 1"
        }
        frame 1001 {
          # "Not Adjustable has a Fixed threshold of 1.25 V"
          # "Trigger AUX"
        }
      }
      n100 = To Unsigned Long Integer(number=w16) -> (unsigned 32bit integer=w56:u32)
      n101 = Boolean To (0,1)(Boolean=w50) -> (0, 1=w49:i16)
      n102 = To Unsigned Long Integer(number=w53) -> (unsigned 32bit integer=w55:u32)
      n103 = call "PicoScopeVoltsToAdc.vi"("Max_adc"="Max ADC value", "Units"=w13, "Range Index"=w14) -> ("ADC count"=w17:i16)
      n104 = dll-call lib="psospa.dll" fn="psospaSetSimpleTrigger" ("ps3000.dll:_ps3000_open_unit@0")(error in=w22, "handle"=w21, "enable"=w49, "source"=w56, "threshold"=w17, "direction"=w55, "delay"=w52, "autoTrigger_us"=w51) -> (error out=w47:errorcluster, "PICO_STATUS"=w48:u32, "handle"=w37:i16)  [unwired: 8 in, 1 out]
      n105 = call "PicoStatus.vi"("PICO STATUS"=w48, "error in"=w47, "source"="psospaSetSimpleTrigger") -> ("error out"=w38:errorcluster)
      n106 = call "PicoErrorHandler2.vi"("error in (no error)"=w38, "handle In"=w37) -> ("error out"=w39:errorcluster)  [unwired: 9 in]
    }
    frame Error {
    }
  }
  "error out" <- w5
  "handle out" <- w6
